vi "Generate image index number.vi"(9 "Minimum Width (4)":i16=4, 11 "FOR loop iteration or existing number of files":i32) -> (3 "Number in string representation (padded with zeroes)":string)   [LabVIEW 2013]
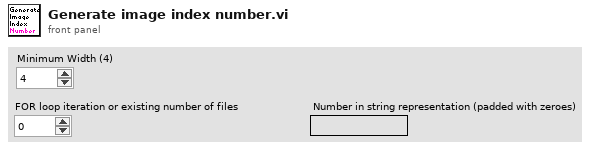
[diagram p1: front panel]
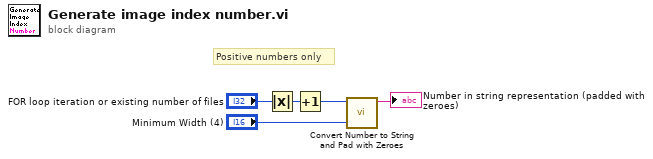
[diagram p0: block diagram]
diagram:
  # "Positive numbers only"
  n1 = Absolute Value(x="FOR loop iteration or existing number of files") -> (abs(x)=w3:i32)
  n2 = Increment(x=w3) -> (x+1=w1:i32)
  n3 = call "Convert Number to String and Pad with Zeroes.vi"("Minimum Width"="Minimum Width (4)", "Number"=w1) -> ("Number in string representation (padded with zeroes)"=→"Number in string representation (padded with zeroes)":string)  [unwired: 9 in]
